vi "Init.vi"(5 "PathControl.lvclass":refnum<class "PathControl.lvclass">, 6 "Environmental classes":refnum<class "Instrument.lvclass">[](array[class]), 7 "XML Handler.lvclass":refnum<class "XML Handler.lvclass">, 8 "error in (no error)":errorcluster, 9 "Instrumentes to Use":T1(array[cluster]), 10 "Device.lvclass":refnum<class "Device.lvclass">, 11 "AM-AM in":refnum<class "AM-AM.lvclass">) -> (0 "error out":errorcluster, 3 "AM-AM out":refnum<class "AM-AM.lvclass">)   [LabVIEW 2020, in "AM-AM.lvclass"]
doc: "Initializes the measurement.\nThis verifies that the instruments are present and adds them into the class data.\nIs also adds the xml handler into the class data."
uses:
  AM-AM.lvclass
  C:/Sandbox/Git_Sandbox/WiSpry Test Framework source code (LV20)/WiSpry Test Framework/Measurements/Measurement.lvclass
  Devices/Device.lvclass
  Instruments/Instrument.lvclass
  XML Handler/XML Handler.lvclass
  Path Control/PathControl.lvclass
  Controls/Init states.ctl
  Instruments/Spectrum Analyzer/Spectrum Analyzer.lvclass
  Instruments/Signal Generator/Signal Generator.lvclass
  Instruments/Power Meter/Power Meter.lvclass
  AM-AM.lvclass/AM-AM.ctl
  Measurement.lvclass/Measurement.ctl
  Devices/Controls/Change setting mode enum.ctl
  Path Control/Measurements Specific Paths.ctl
  Devices/PIC-device/PIC-Device.lvclass
  Measurement.lvclass
panel:
  out "Current State":string
  out "Initializing AM-AM Measurement":u8(slide) scale=0.0..100.0
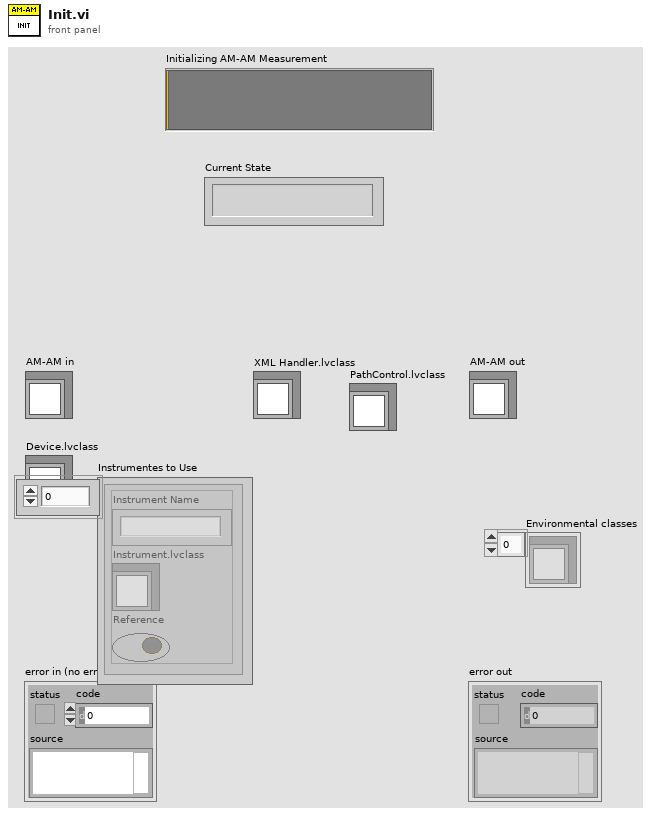
[diagram p1: front panel]
types:
  T1 = cluster{"Instrument Name":string, "Instrument.lvclass":refnum<class "Instrument.lvclass">, "Reference":bool}[]
  T2 = typedef "AM-AM.lvclass/Init states.ctl" = enum16{"Verify instruments", "Init Sweep Parameters", "Init Instruments", "Add Device", "Init Device", "Create test in XML", "Set path", "Done"}
  T3 = typedef "PIC-Device.lvclass/Change setting mode enum.ctl" = enum16{"Init", "Next", "Reset"}
  T4 = typedef "PathControl.lvclass/Measurements Specific Paths.ctl" = enum16{"No calibration", "Harmonics", "IMD", "S Parameter", "AM-AM", "MCCW-ACLR", "DC", "LCR", "Power Meter GUI", "RF Power"}
  T5 = typedef "AM-AM.lvclass/Config info.ctl" = cluster{"RBW":dbl, "VBW ":dbl, "Number of Averages":dbl, "Average On":bool, "Power":cluster{"Cluster ":cluster{"From":dbl, "To":dbl, "Step":dbl}, "Array":dbl[], "Use Array":bool}, "Frequency":cluster{"Cluster ":cluster{"From":dbl, "To":dbl, "Step":dbl}, "Array":dbl[], "Use Array":bool}, "Loop order":T6, "Power Window":dbl}
  T6 = typedef "AM-AM.lvclass/Loop order.ctl" = enum16{"Device -> Power -> Frequency", "Device -> Frequency -> Power"}
  T7 = cluster{"Cluster ":cluster{"From":dbl, "To":dbl, "Step":dbl}, "Array":dbl[], "Use Array":bool}
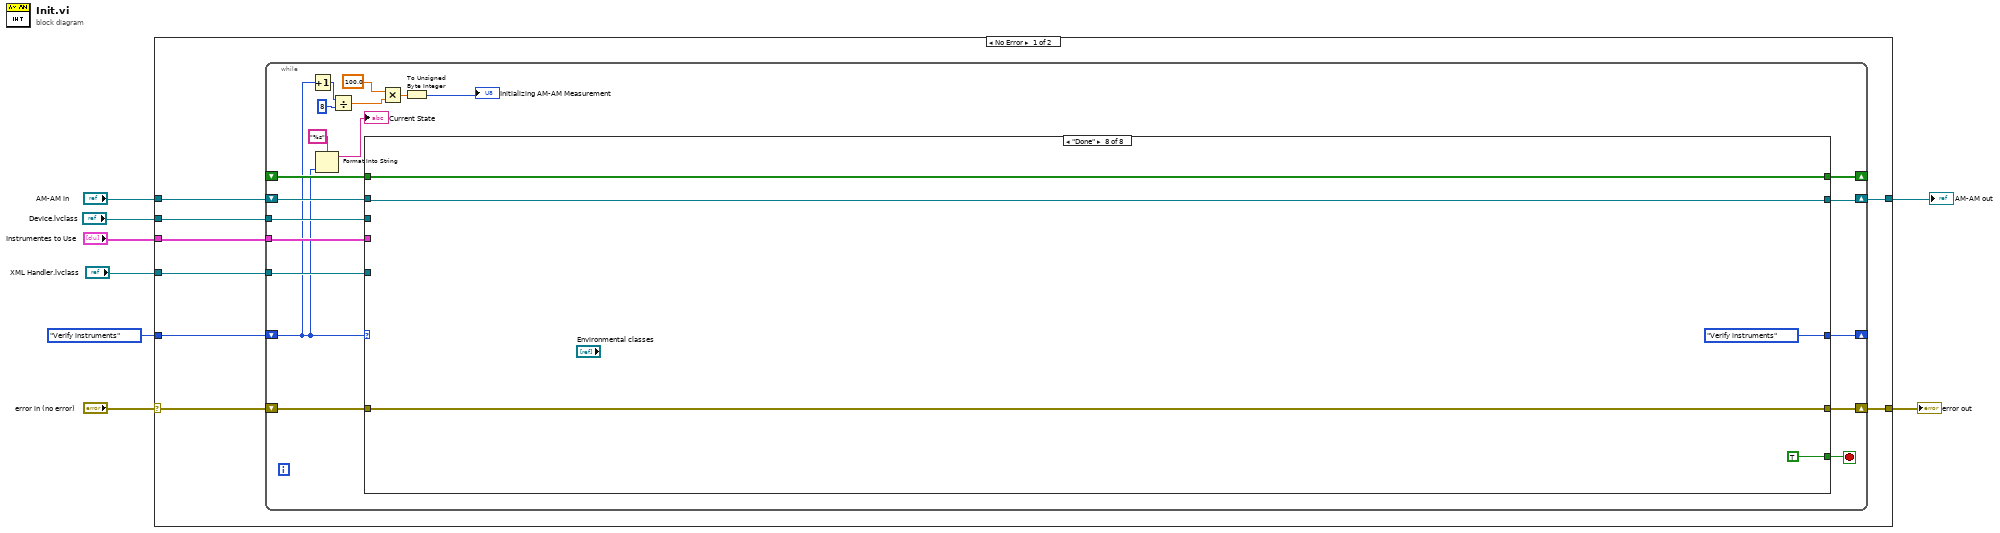
[diagram p0: block diagram]
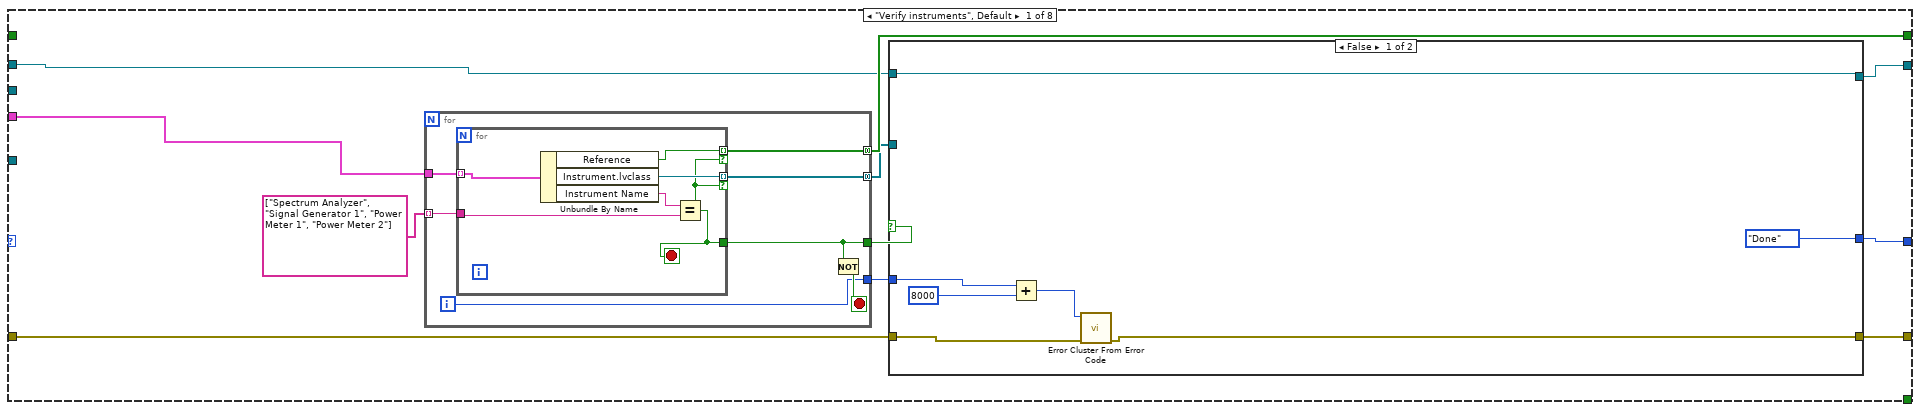
[diagram p2: hidden frame]
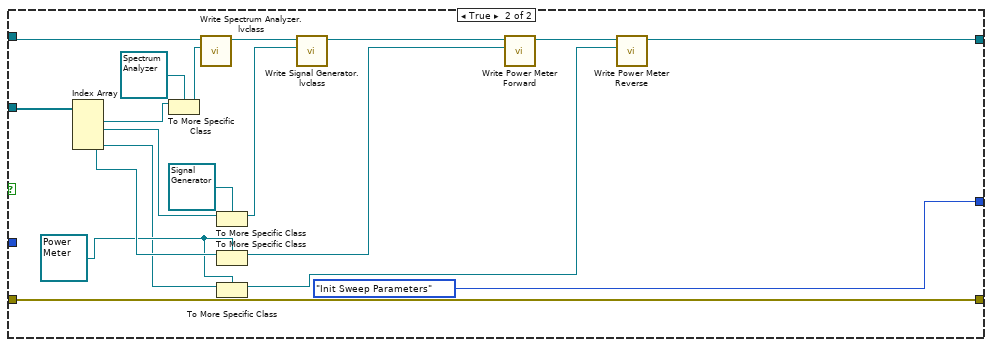
[diagram p3: hidden frame]
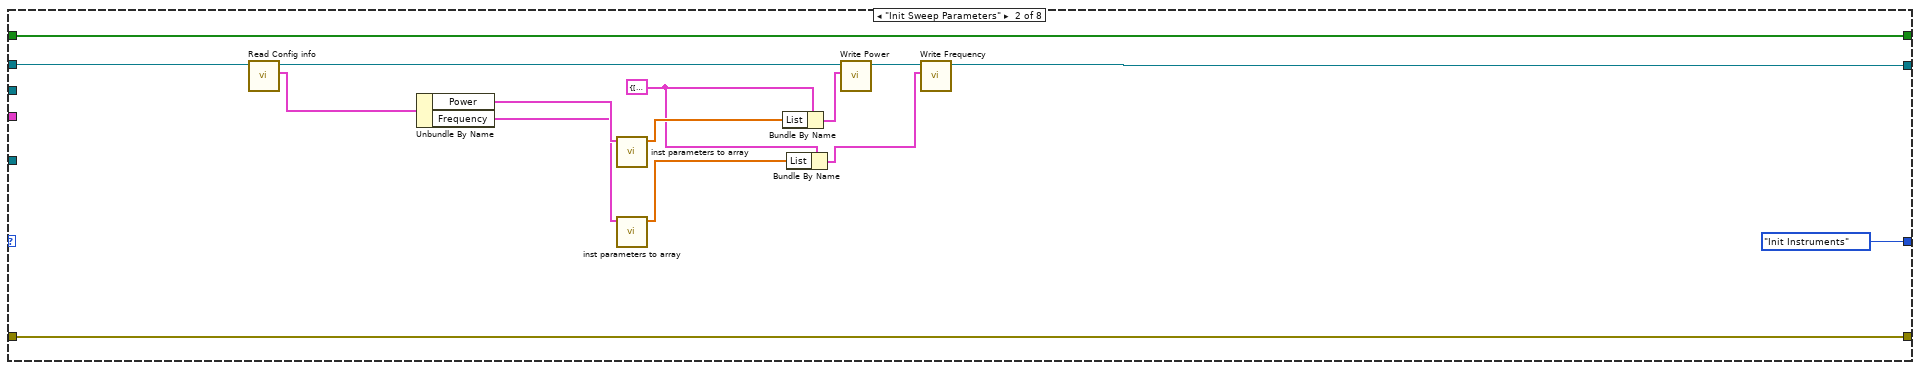
[diagram p4: hidden frame]
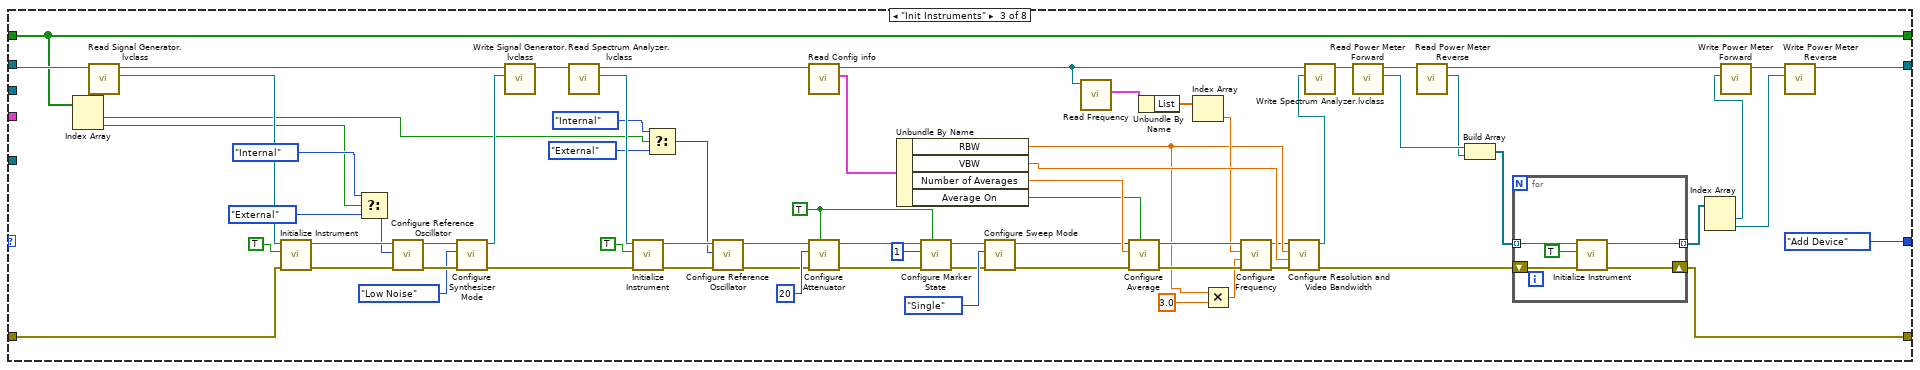
[diagram p5: hidden frame]
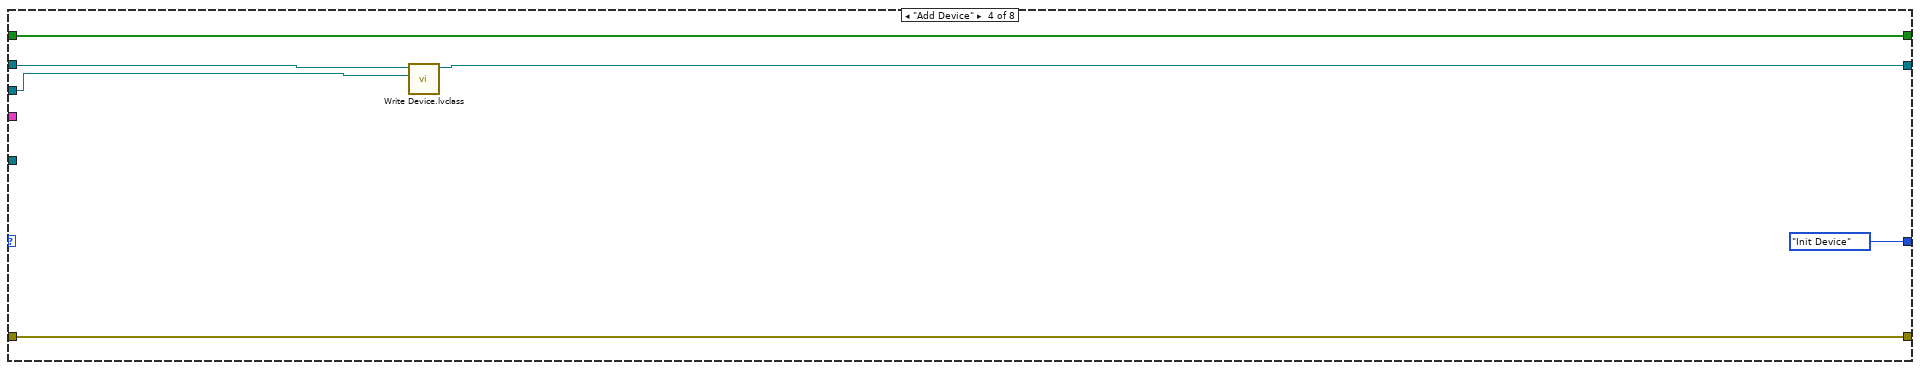
[diagram p6: hidden frame]
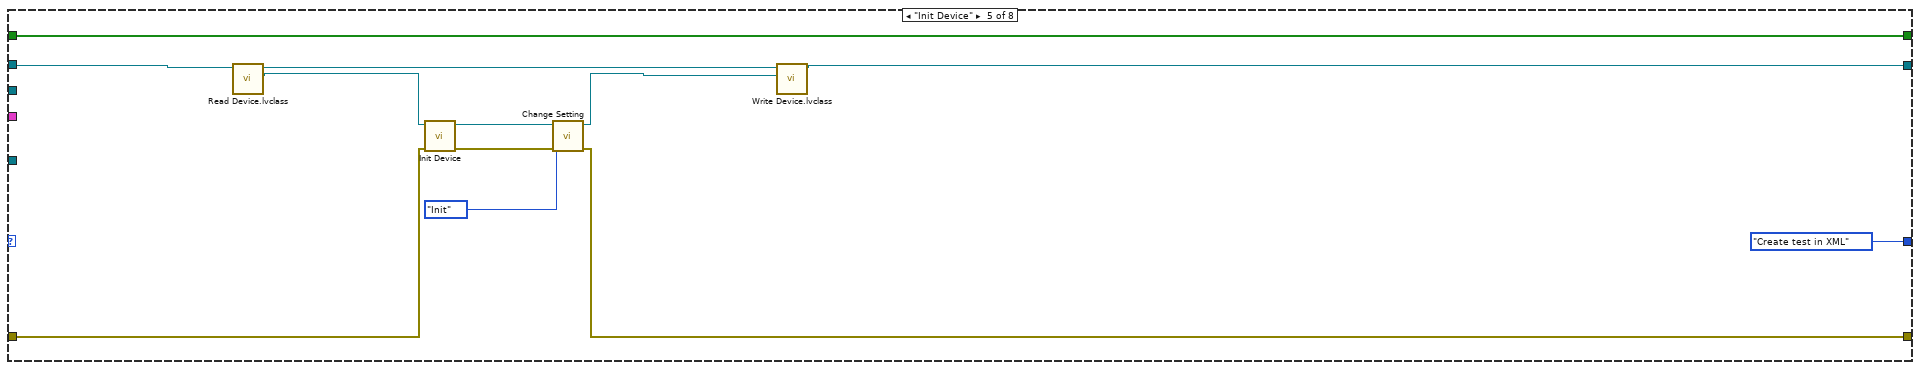
[diagram p7: hidden frame]
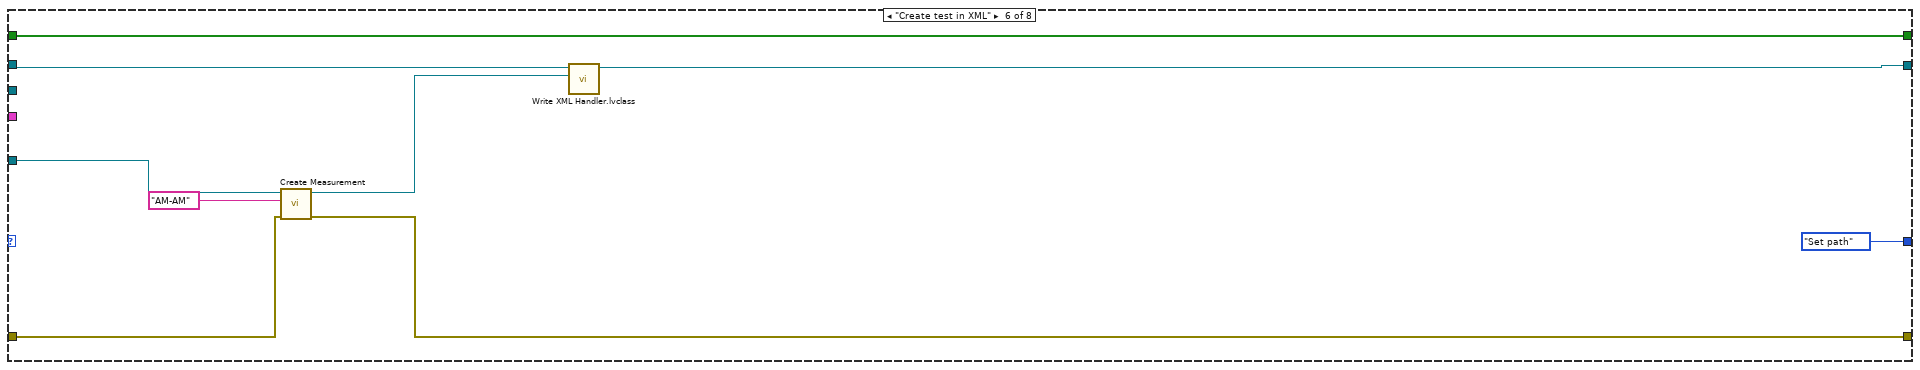
[diagram p8: hidden frame]
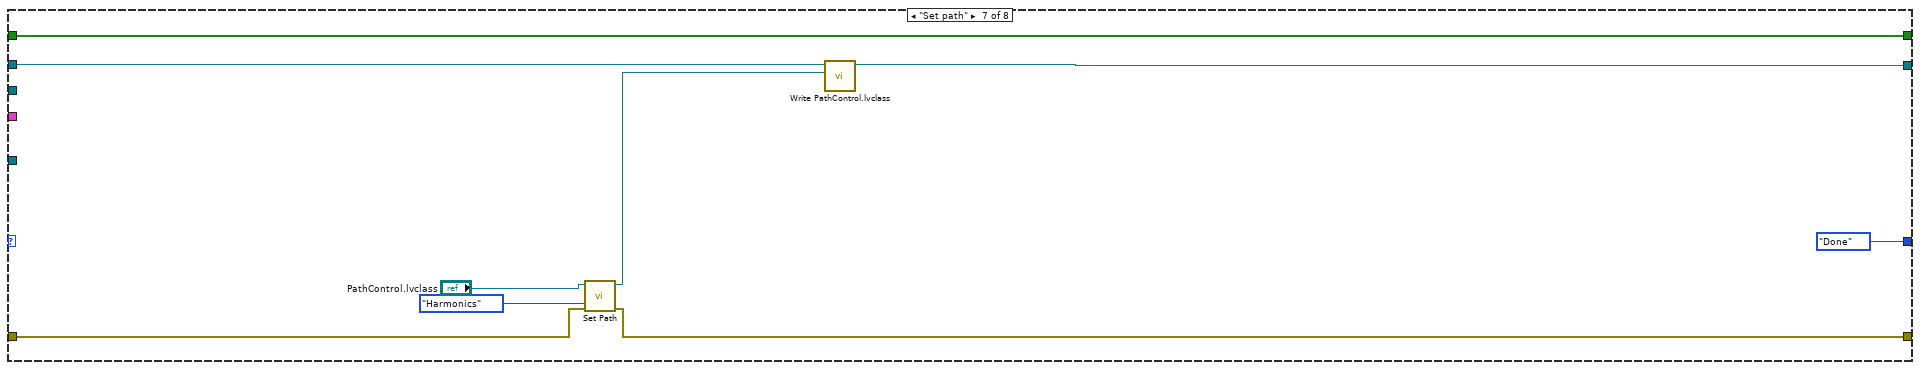
[diagram p9: hidden frame]
diagram:
  n1 = case shown="No Error" "error in (no error)" {
    selector: "error in (no error)" -> [w16 w217]
    tunnel: "Instrumentes to Use" -> [w15 _]
    tunnel: "Device.lvclass" -> [w14 _]
    tunnel: "AM-AM in" -> [w13 w218]
    tunnel: Init_states."Verify instruments" -> [w12 _]
    tunnel: [w11 w217] -> w3
    tunnel: [w10 w218] -> w2
    tunnel: "XML Handler.lvclass" -> [w9 _]
    frame No Error {
      n2 = while {
        shift-right: [w31] -> w11
        shift-left: w16 -> [w32]
        tunnel: w15 -> [w36]
        tunnel: w14 -> [w33]
        shift-right: [w34] -> w10
        shift-left: w13 -> [w35]
        shift-right: [w28] -> _
        shift-left: w12 -> [w23]
        tunnel: w9 -> [w29]
        shift-right: [w27] -> _
        shift-left: _ -> [w26]
        stop <- w30 stop-if-true
        n3 = Increment(x=w23) -> (x+1=w22:T2)
        n4 = Format Into String(format string="%s", w23) -> (resulting string=→"Current State":string)  [unwired: 2 in, 1 out]
        n5 = Divide(x=w22, y=8) -> (x/y=w20:dbl)
        n6 = case shown="\"Done\"" w23 {
          tunnel: w36 -> [w47 _ _ _ _ _ _ _]
          tunnel: w35 -> [w37 w99 w170 w181 w187 w200 w210 w212]
          tunnel: [w46 w93 w105 w180 w185 w196 w211 w212] -> w34
          tunnel: w33 -> [_ _ _ w179 _ _ _ _]
          tunnel: w32 -> [w45 w100 w167 w177 w193 w198 w207 w214]
          tunnel: [w44 w100 w112 w177 w189 w197 w206 w214] -> w31
          tunnel: [w43 Init_states."Init Instruments" Init_states."Add Device" Init_states."Init Device" Init_states."Create test in XML" Init_states."Set path" Init_states."Done" Init_states."Verify instruments"] -> w28
          tunnel: [_ _ _ _ _ _ _ TRUE] -> w30
          tunnel: w29 -> [_ _ _ _ _ w202 _ _]
          tunnel: [w42 w87 w148 w176 w182 w194 w203 w216] -> w27
          tunnel: w26 -> [_ w87 w148 w176 w182 w194 w203 w216]
          frame "Verify instruments", Default {
            n7 = for {
              tunnel: w47 -> [w80]
              tunnel: string[] ["Spectrum Analyzer", "Signal Generator 1", "Power Meter 1", "Power Meter 2"] -> [w76] mode=indexing
              tunnel: [w79] -> w39 mode=concatenating
              tunnel: [w78] -> w40
              tunnel: [w75] -> w38
              tunnel: [w74] -> w42 mode=concatenating
              i -> [w75]
              stop <- w77 stop-if-true
              n8 = for {
                tunnel: w80 -> [w86] mode=indexing
                tunnel: w76 -> [w84]
                tunnel: [w83] -> w79 mode=indexing if=w81
                tunnel: [w81] -> w78
                tunnel: [w82] -> w74 mode=indexing if=w81
                stop <- w81 stop-if-true
                n9 = Unbundle By Name(w86) -> ("Reference"=w82:bool, "Instrument.lvclass"=w83:refnum<class "Instrument.lvclass">, "Instrument Name"=w85:string)
                n10 = Equal?(x=w85, y=w84) -> (x = y?=w81:bool)
              }
              n11 = Not(x=w78) -> (.not. x?=w77:bool)
            }
            n12 = case shown="False" w40 {
              tunnel: w39 -> [_ w71]
              tunnel: w37 -> [w54 w73]
              tunnel: [w54 w58] -> w46
              tunnel: w45 -> [w53 w63]
              tunnel: w38 -> [w52 _]
              tunnel: [w49 w63] -> w44
              tunnel: [Init_states."Done" Init_states."Init Sweep Parameters"] -> w43
              frame False {
                n13 = Add(x=w52, y=8000) -> (x+y=w50:i32)
                n14 = call <vilib>:"Error Cluster From Error Code.vi"("error in (no error)"=w53, "error code (0)"=w50) -> ("error out"=w49:errorcluster)  [unwired: 7 in]
              }
              frame True {
                w57 = refnum<class "Power Meter.lvclass"> refnum ("Power Meter.lvclass")
                n15 = Index Array(array=w71) -> (element #1=w70:refnum<class "Instrument.lvclass">, element #2=w67:refnum<class "Instrument.lvclass">, element #3=w61:refnum<class "Instrument.lvclass">, element #4=w56:refnum<class "Instrument.lvclass">)  [unwired: 4 in]
                n16 = To More Specific Class(target class=refnum<class "Spectrum Analyzer.lvclass"> refnum ("Spectrum Analyzer.lvclass"), reference=w70) -> (specific class reference=w69:refnum<class "Spectrum Analyzer.lvclass">)  [unwired: 1 in, 1 out]
                n17 = call "Write Spectrum Analyzer.lvclass.vi"("Spectrum Analyzer.lvclass"=w69, "AM-AM in"=w73) -> ("AM-AM out"=w72:refnum<class "AM-AM.lvclass">)  [unwired: 9 in]
                n18 = To More Specific Class(target class=refnum<class "Signal Generator.lvclass"> refnum ("Signal Generator.lvclass"), reference=w67) -> (specific class reference=w65:refnum<class "Signal Generator.lvclass">)  [unwired: 1 in, 1 out]
                n19 = To More Specific Class(target class=w57, reference=w61) -> (specific class reference=w60:refnum<class "Power Meter.lvclass">)  [unwired: 1 in, 1 out]
                n20 = To More Specific Class(target class=w57, reference=w56) -> (specific class reference=w55:refnum<class "Power Meter.lvclass">)  [unwired: 1 in, 1 out]
                n21 = call "Write Signal Generator.lvclass.vi"("Signal Generator.lvclass"=w65, "AM-AM in"=w72) -> ("AM-AM out"=w62:refnum<class "AM-AM.lvclass">)  [unwired: 9 in]
                n22 = call "Write Power Meter Forward.vi"("Power Meter Forward"=w60, "AM-AM in"=w62) -> ("AM-AM out"=w59:refnum<class "AM-AM.lvclass">)  [unwired: 9 in]
                n23 = call "Write Power Meter Reverse.vi"("Power Meter.lvclass"=w55, "AM-AM in"=w59) -> ("AM-AM out"=w58:refnum<class "AM-AM.lvclass">)  [unwired: 9 in]
              }
            }
          }
          frame "Init Sweep Parameters" {
            w91 = cluster{"List":dbl[], "Index":i32, "Last":bool} {"List"=[], "Index"=0, "Last"=FALSE} ("Power")
            n24 = call "Read Config info.vi"("AM-AM in"=w99) -> ("Config info"=w98:T5, "AM-AM out"=w95:refnum<class "AM-AM.lvclass">)  [unwired: 9 in]
            n25 = Unbundle By Name(w98) -> ("Power"=w97:T7, "Frequency"=w96:T7)
            n26 = call "inst parameters to array.vi"("Input"=w97) -> ("Array"=w92:dbl[])  [unwired: 10 in]
            n27 = call "inst parameters to array.vi"("Input"=w96) -> ("Array"=w89:dbl[])  [unwired: 10 in]
            n28 = Bundle By Name(cluster=w91, "List"=w92) -> (w90:cluster{"List":dbl[], "Index":i32, "Last":bool})
            n29 = Bundle By Name(cluster=w91, "List"=w89) -> (w88:cluster{"List":dbl[], "Index":i32, "Last":bool})
            n30 = call "Write Power.vi"("Power"=w90, "AM-AM in"=w95) -> ("AM-AM out"=w94:refnum<class "AM-AM.lvclass">)  [unwired: 9 in]
            n31 = call "Write Frequency.vi"("Frequency"=w88, "AM-AM in"=w94) -> ("AM-AM out"=w93:refnum<class "AM-AM.lvclass">)  [unwired: 9 in]
          }
          frame "Init Instruments" {
            w153 = TRUE ("Auto Attenuator (T)")
            n32 = Index Array(array=w148) -> (element #1=w129:bool, element #2=w130:bool)  [unwired: 2 in]
            n33 = call "Read Signal Generator.lvclass.vi"("AM-AM in"=w170) -> ("Signal Generator.lvclass"=w169:refnum<class "Signal Generator.lvclass">, "AM-AM out"=w166:refnum<class "AM-AM.lvclass">)  [unwired: 9 in]
            n34 = call-dynamic "Initialize Instrument.vi"("error in (no error)"=w167, "Reset"=TRUE, "Instrument in"=w169) -> ("error out"=w142:errorcluster, "Instrument out"=w147:refnum<class "Signal Generator.lvclass">)  [unwired: 7 in]
            n35 = Select(t=enum16{"Internal", "External"}."Internal" ("Reference Mode"), s=w130, f=enum16{"Internal", "External"}."External") -> (s? t:f=w144:enum16{"Internal", "External"})
            n36 = call-dynamic "Configure Reference Oscillator.vi"("error in (no error)"=w142, "Reference Mode"=w144, "Signal Generator in"=w147) -> ("error out"=w143:errorcluster, "Signal Generator out"=w141:refnum<class "Signal Generator.lvclass">)  [unwired: 7 in]
            n37 = call-dynamic "Configure Synthesizer Mode.vi"("error in (no error)"=w143, "Synthesizer Mode"=enum16{"Normal", "Low Noise"}."Low Noise", "Signal Generator in"=w141) -> ("error out"=w139:errorcluster, "Signal Generator out"=w131:refnum<class "Signal Generator.lvclass">)  [unwired: 7 in]
            n38 = call "Write Signal Generator.lvclass.vi"("Signal Generator.lvclass"=w131, "AM-AM in"=w166) -> ("AM-AM out"=w165:refnum<class "AM-AM.lvclass">)  [unwired: 9 in]
            n39 = call "Read Spectrum Analyzer.lvclass.vi"("AM-AM in"=w165) -> ("Spectrum Analyzer.lvclass"=w164:refnum<class "Spectrum Analyzer.lvclass">, "AM-AM out"=w160:refnum<class "AM-AM.lvclass">)  [unwired: 9 in]
            n40 = call-dynamic "Initialize Instrument.vi"("error in (no error)"=w139, "Reset"=TRUE, "Instrument in"=w164) -> ("error out"=w138:errorcluster, "Instrument out"=w137:refnum<class "Spectrum Analyzer.lvclass">)  [unwired: 7 in]
            n41 = Select(t=enum16{"Internal", "External"}."Internal" ("Reference Mode"), s=w129, f=enum16{"Internal", "External"}."External") -> (s? t:f=w133:enum16{"Internal", "External"})
            n42 = call-dynamic "Configure Reference Oscillator.vi"("error in (no error)"=w138, "Reference Oscillator (Internal)"=w133, "Spectrum Analyzer in"=w137) -> ("error out"=w135:errorcluster, "Spectrum Analyzer out"=w136:refnum<class "Spectrum Analyzer.lvclass">)  [unwired: 7 in]
            n43 = call "Read Config info.vi"("AM-AM in"=w160) -> ("Config info"=w159:T5, "AM-AM out"=w126:refnum<class "AM-AM.lvclass">)  [unwired: 9 in]
            n44 = call-dynamic "Configure Attenuator.vi"("Auto Attenuator (T)"=w153, "error in (no error)"=w135, "Attenuator (dB)"=u32 20, "Spectrum Analyzer in"=w136) -> ("error out"=w155:errorcluster, "Spectrum Analyzer out"=w154:refnum<class "Spectrum Analyzer.lvclass">)  [unwired: 6 in]
            n45 = Unbundle By Name(w159) -> ("RBW"=w122:dbl, "VBW"=w158:dbl, "Number of Averages"=w157:dbl, "Average On"=w156:bool)
            n46 = call-dynamic "Configure Marker State.vi"("Maker On (F)"=w153, "error in (no error)"=w155, "Marker Number (1)"=u32 1, "Spectrum Analyzer in"=w154) -> ("error out"=w149:errorcluster, "Spectrum Analyzer out"=w150:refnum<class "Spectrum Analyzer.lvclass">)  [unwired: 6 in]
            n47 = call-dynamic "Configure Sweep Mode.vi"("error in (no error)"=w149, "Sweep Mode"=enum16{"Continuous", "Single"}."Single", "Spectrum Analyzer in"=w150) -> ("error out"=w117:errorcluster, "Spectrum Analyzer out"=w118:refnum<class "Spectrum Analyzer.lvclass">)  [unwired: 7 in]
            n48 = call "Read Frequency.vi"("AM-AM in"=w126) -> ("Frequency"=w125:cluster{"List":dbl[], "Index":i32, "Last":bool})  [unwired: 9 in, 1 out]
            n49 = call-dynamic "Configure Average.vi"("Average On (F)"=w156, "error in (no error)"=w117, "Average"=w157, "Spectrum Analyzer in"=w118) -> ("error out"=w128:errorcluster, "Spectrum Analyzer out"=w127:refnum<class "Spectrum Analyzer.lvclass">)  [unwired: 6 in]
            n50 = Unbundle By Name(w125) -> ("List"=w124:dbl[])
            n51 = Index Array(array=w124) -> (element=w123:dbl)  [unwired: 1 in]
            n52 = Multiply(x=w122, y=3.0) -> (x*y=w120:dbl)
            n53 = call-dynamic "Configure Frequency.vi"("error in (no error)"=w128, "Span/Stop Frequency [Hz]"=w120, "Center/Start Frequency [Hz]"=w123, "Spectrum Analyzer in"=w127) -> ("error out"=w115:errorcluster, "Spectrum Analyzer out"=w116:refnum<class "Spectrum Analyzer.lvclass">)  [unwired: 6 in]
            n54 = call-dynamic "Configure Resolution and Video Bandwidth.vi"("error in (no error)"=w115, "VBW [Hz]"=w158, "RBW [Hz]"=w122, "Spectrum Analyzer in"=w116) -> ("error out"=w113:errorcluster, "Spectrum Analyzer out"=w114:refnum<class "Spectrum Analyzer.lvclass">)  [unwired: 6 in]
            n55 = call "Write Spectrum Analyzer.lvclass.vi"("Spectrum Analyzer.lvclass"=w114, "AM-AM in"=w126) -> ("AM-AM out"=w119:refnum<class "AM-AM.lvclass">)  [unwired: 9 in]
            n56 = call "Read Power Meter Forward.vi"("AM-AM in"=w119) -> ("Power Meter Forward"=w109:refnum<class "Power Meter.lvclass">, "AM-AM out"=w111:refnum<class "AM-AM.lvclass">)  [unwired: 9 in]
            n57 = call "Read Power Meter Reverse.vi"("AM-AM in"=w111) -> ("Power Meter.lvclass"=w108:refnum<class "Power Meter.lvclass">, "AM-AM out"=w110:refnum<class "AM-AM.lvclass">)  [unwired: 9 in]
            n58 = Build Array(w109, w108) -> (w107:refnum<class "Power Meter.lvclass">[])
            n59 = for {
              shift-right: [w173] -> w112
              shift-left: w113 -> [w175]
              tunnel: w107 -> [w172] mode=indexing
              tunnel: [w171] -> w104 mode=indexing
              n60 = call-dynamic "Initialize Instrument.vi"("error in (no error)"=w175, "Reset"=TRUE, "Instrument in"=w172) -> ("error out"=w173:errorcluster, "Instrument out"=w171:refnum<class "Power Meter.lvclass">)  [unwired: 7 in]
            }
            n61 = Index Array(array=w104) -> (element #1=w103:refnum<class "Power Meter.lvclass">, element #2=w102:refnum<class "Power Meter.lvclass">)  [unwired: 2 in]
            n62 = call "Write Power Meter Forward.vi"("Power Meter Forward"=w103, "AM-AM in"=w110) -> ("AM-AM out"=w106:refnum<class "AM-AM.lvclass">)  [unwired: 9 in]
            n63 = call "Write Power Meter Reverse.vi"("Power Meter.lvclass"=w102, "AM-AM in"=w106) -> ("AM-AM out"=w105:refnum<class "AM-AM.lvclass">)  [unwired: 9 in]
          }
          frame "Add Device" {
            n64 = call "Write Device.lvclass.vi"("Device.lvclass"=w179, "Measurements in"=w181) -> ("Measurements out"=w180:refnum<class "AM-AM.lvclass">)  [unwired: 9 in]
          }
          frame "Init Device" {
            n65 = call "Read Device.lvclass.vi"("Measurements in"=w187) -> ("Device.lvclass"=w186:refnum<class "Device.lvclass">, "Measurements out"=w184:refnum<class "AM-AM.lvclass">)  [unwired: 9 in]
            n66 = call-dynamic "Init Device.vi"("error in (no error)"=w193, "Device in"=w186) -> ("error out"=w191:errorcluster, "Device out"=w192:refnum<class "Device.lvclass">)  [unwired: 8 in]
            n67 = call-dynamic "Change Setting.vi"("error in (no error)"=w191, "Change setting mode"=Change_setting_mode_enum."Init", "Device in"=w192) -> ("error out"=w189:errorcluster, "Device out"=w183:refnum<class "Device.lvclass">)  [unwired: 5 in, 2 out]
            n68 = call "Write Device.lvclass.vi"("Device.lvclass"=w183, "Measurements in"=w184) -> ("Measurements out"=w185:refnum<class "AM-AM.lvclass">)  [unwired: 9 in]
          }
          frame "Create test in XML" {
            n69 = call "Create Measurement.vi"("error in (no error)"=w198, "Measurement Name"="AM-AM", "XML Handler in"=w202) -> ("error out"=w197:errorcluster, "XML Handler out"=w199:refnum<class "XML Handler.lvclass">)  [unwired: 7 in]
            n70 = call "Write XML Handler.lvclass.vi"("XML Handler.lvclass"=w199, "Measurements in"=w200) -> ("Measurements out"=w196:refnum<class "AM-AM.lvclass">)  [unwired: 9 in]
          }
          frame "Set path" {
            n71 = call "Set Path.vi"("error in (no error)"=w207, "Measurement specfic paths"=Measurements_Specific_Paths."Harmonics", "PathControl in"="PathControl.lvclass") -> ("error out"=w206:errorcluster, "PathControl out"=w205:refnum<class "PathControl.lvclass">)  [unwired: 7 in]
            n72 = call "Write PathControl.lvclass.vi"("PathControl.lvclass"=w205, "Measurements in"=w210) -> ("Measurements out"=w211:refnum<class "AM-AM.lvclass">)  [unwired: 9 in]
          }
          frame "Done" {
          }
        }
        n73 = Multiply(x=100.0 ("y"), y=w20) -> (x*y=w18:dbl)
        n74 = To Unsigned Byte Integer(number=w18) -> (unsigned 8bit integer=→"Initializing AM-AM Measurement":u8)
      }
    }
    frame Error {
    }
  }
  "error out" <- w3
  "AM-AM out" <- w2
